vi "~sequence2.vi"(6 "i":i32, 10 "Array":T5[](array[typedef])) -> (0 "Command":string, 1 "Attenuation dB":dbl, 2 "Phase Shift deg":dbl, 3 "NewSetup":T1, 4 "Sequence is done":bool)   [LabVIEW 2017]
uses:
  Classes/Sequence/SequenceSubvis/TestStep-StepType.ctl
  Classes/Sequence/SequenceSubvis/RF Direction.ctl
  Classes/Sequence/SequenceSubvis/PolarizationSelect.ctl
  Classes/Sequence/SequenceSubvis/TestStepTypes.ctl
  Classes/Sequence/SequenceSubvis/TestStep.ctl
  Classes/Sequence/SequenceSubvis/PatchNewTestStep.ctl
panel:
  out "Test":T4
  # "This oject has members:\n- init\n- sequence\n- reset ?"
  # "NewStep\nNextPhaseShift\nNextAtten\nSequenceComplete"
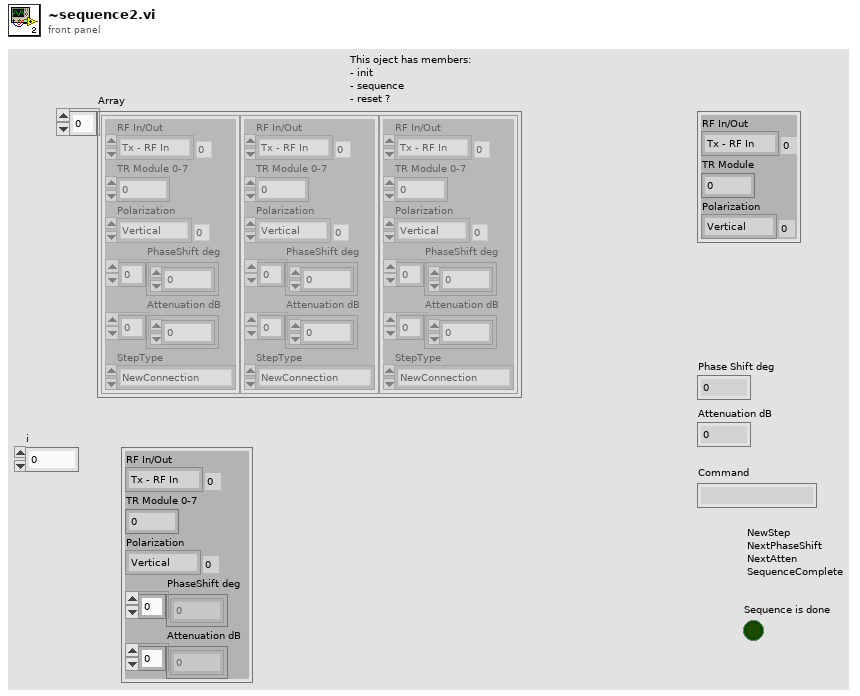
[diagram p1: front panel]
types:
  T1 = typedef "PatchNewTestStep.ctl" = cluster{"RF In/Out":T2, "TR Module":i32, "Polarization":T3}
  T2 = typedef "RF Direction.ctl" = enum16{"Tx - RF In", "Rx - RF Out"}
  T3 = typedef "PolarizationSelect.ctl" = enum16{"Vertical", "Horizontal"}
  T4 = typedef "TestStep.ctl" = cluster{"RF In/Out":T2, "TR Module 0-7":i32, "Polarization":T3, "PhaseShift deg":dbl[], "Attenuation dB":dbl[]}
  T5 = typedef "TestStep-StepType.ctl" = cluster{"RF In/Out":T2, "TR Module 0-7":i32, "Polarization":T3, "PhaseShift deg":dbl[], "Attenuation dB":dbl[], "StepType":T6}
  T6 = typedef "TestStepTypes.ctl" = enum16{"NewConnection", "SweepTest", "Motion", "Finish"}
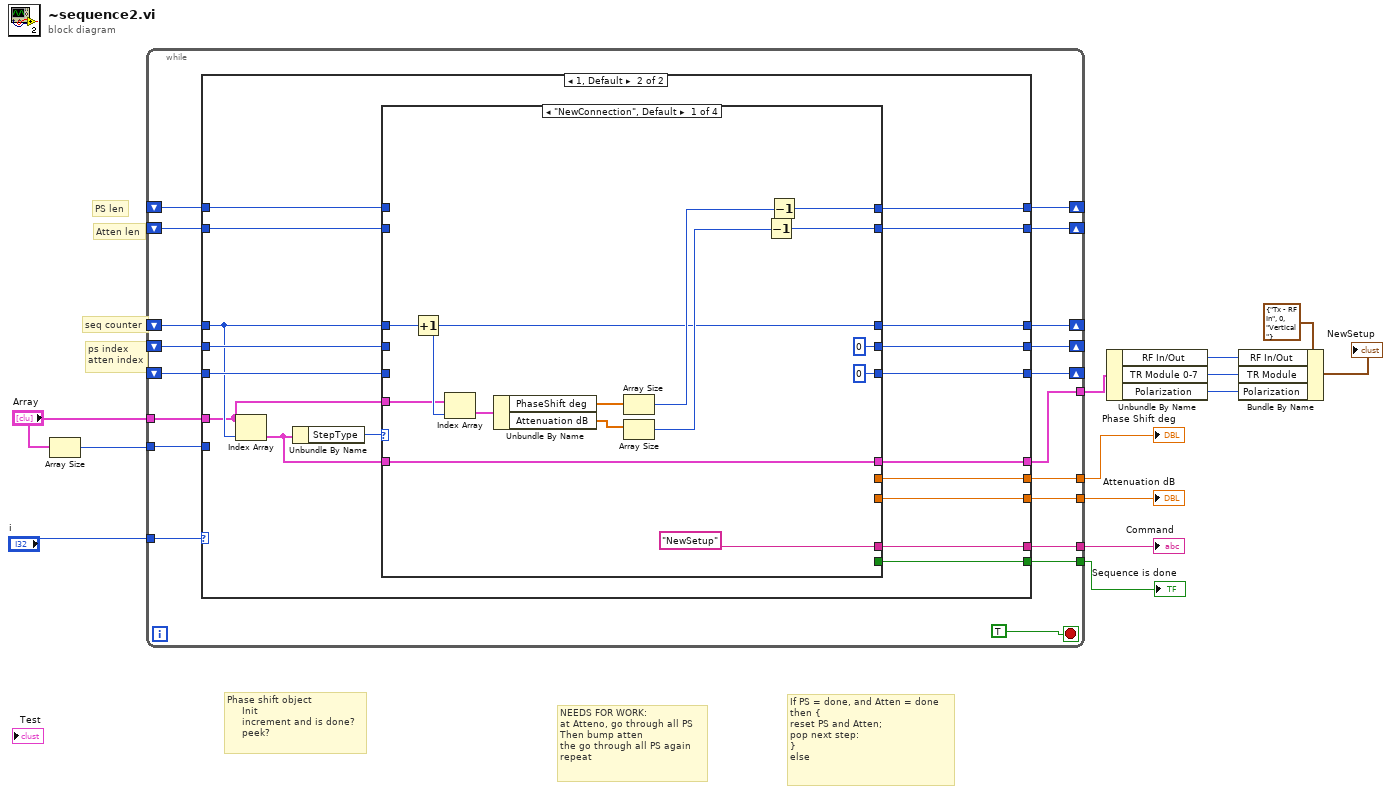
[diagram p0: block diagram]
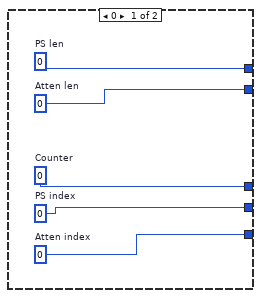
[diagram p2: hidden frame]
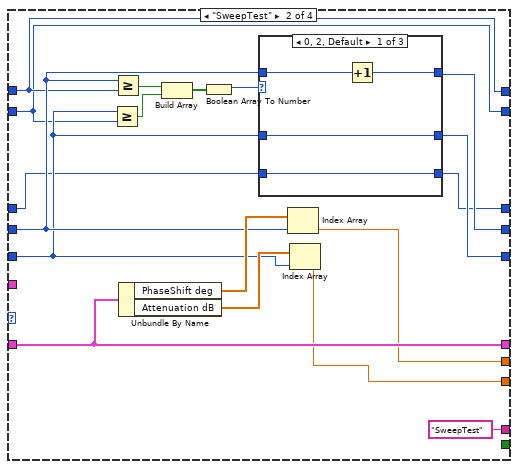
[diagram p3: hidden frame]
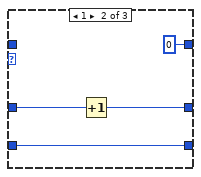
[diagram p4: hidden frame]
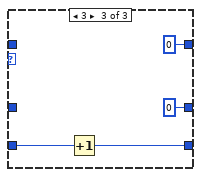
[diagram p5: hidden frame]
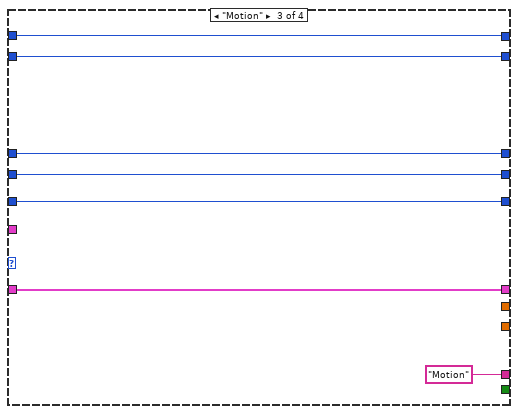
[diagram p6: hidden frame]
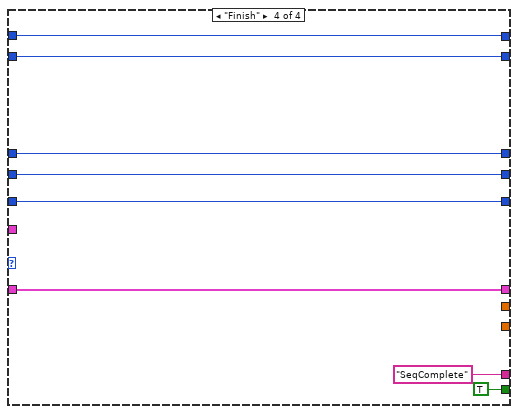
[diagram p7: hidden frame]
diagram:
  # "ps index\natten index"
  # "seq counter"
  # "Atten len"
  # "PS len"
  # "NEEDS FOR WORK:\nat Atteno, go through all PS\nThen bump atten\nthe go through all PS again\nrepeat"
  # "If PS = done, and Atten = done\nthen {\nreset PS and Atten;\npop next step:\n}\nelse"
  # "Phase shift object\n     Init\n     increment and is done?\n     peek?"
  n1 = Array Size(array="Array") -> (size(s)=w11:i32)
  n2 = while {
    shift-right: [w30] -> _
    shift-left: _ -> [w21]
    tunnel: "Array" -> [w29]
    shift-right: [w32] -> _
    shift-left: _ -> [w25]
    shift-right: [w31] -> _
    shift-left: _ -> [w24]
    shift-right: [w28] -> _
    shift-left: _ -> [w23]
    shift-right: [w27] -> _
    shift-left: _ -> [w22]
    tunnel: w11 -> [w20]
    tunnel: "i" -> [w19]
    tunnel: [w18] -> w5
    tunnel: [w17] -> w4
    tunnel: [w16] -> w3
    tunnel: [w15] -> w2
    tunnel: [w14] -> w1
    stop <- TRUE stop-if-true
    n3 = case shown="1, Default" w19 {
      tunnel: [w34 w44] -> w32
      tunnel: [w33 w45] -> w31
      tunnel: [w35 w40] -> w30
      tunnel: w29 -> [_ w38]
      tunnel: [w36 w42] -> w28
      tunnel: [w37 w43] -> w27
      tunnel: w25 -> [_ w51]
      tunnel: w24 -> [_ w50]
      tunnel: w23 -> [_ w46]
      tunnel: w22 -> [_ w47]
      tunnel: w21 -> [_ w41]
      tunnel: w20 -> [_ _]
      tunnel: [_ w53] -> w18
      tunnel: [_ w52] -> w17
      tunnel: [_ w49] -> w16
      tunnel: [_ w48] -> w15
      tunnel: [_ w39] -> w14
      frame 0 {
        w37 = 0  # PS len
        w36 = 0  # Atten len
        w33 = 0  # Atten index
        w34 = 0  # PS index
        w35 = 0  # Counter
      }
      frame 1, Default {
        n4 = Index Array(array=w38, index=w41) -> (element=w54:T5)
        n5 = Unbundle By Name(w54) -> ("StepType"=w55:T6)
        n6 = case shown="\"NewConnection\", Default" w55 {
          tunnel: w54 -> [w59 w86 w100 w108]
          tunnel: ["NewSetup" ("Command") "SweepTest" ("Command") "Motion" ("Command") "SeqComplete" ("Command")] -> w53
          tunnel: [w59 w86 w100 w108] -> w52
          tunnel: w51 -> [_ w77 w102 w110]
          tunnel: w50 -> [_ w76 w101 w109]
          tunnel: [_ w83 _ _] -> w49
          tunnel: [_ w82 _ _] -> w48
          tunnel: w47 -> [_ w73 w105 w113]
          tunnel: w46 -> [_ w72 w104 w112]
          tunnel: [0 ("Atten index") w75 w101 w109] -> w45
          tunnel: [0 w74 w102 w110] -> w44
          tunnel: [w57 w73 w105 w113] -> w43
          tunnel: [w56 w72 w104 w112] -> w42
          tunnel: w41 -> [w64 w70 w103 w111]
          tunnel: [w60 w71 w103 w111] -> w40
          tunnel: [_ _ _ TRUE] -> w39
          tunnel: w38 -> [w58 _ _ _]
          frame "NewConnection", Default {
            n7 = Increment(x=w64) -> (x+1=w60:i32)
            n8 = Index Array(array=w58, index=w60) -> (element=w61:T5)
            n9 = Unbundle By Name(w61) -> ("PhaseShift deg"=w68:dbl[], "Attenuation dB"=w67:dbl[])
            n10 = Array Size(array=w68) -> (size(s)=w66:i32)
            n11 = Array Size(array=w67) -> (size(s)=w65:i32)
            n12 = Decrement(x=w65) -> (x-1=w56:i32)
            n13 = Decrement(x=w66) -> (x-1=w57:i32)
          }
          frame "SweepTest" {
            n14 = Greater Or Equal?(x=w76, y=w72) -> (x >= y?=w80:bool)
            n15 = Greater Or Equal?(x=w77, y=w73) -> (x >= y?=w81:bool)
            n16 = Unbundle By Name(w86) -> ("PhaseShift deg"=w85:dbl[], "Attenuation dB"=w84:dbl[])
            n17 = Build Array(w81, w80) -> (w79:bool[])
            n18 = Boolean Array To Number(Boolean array=w79) -> (number=w78:u32)
            n19 = case shown="0, 2, Default" w78 {
              tunnel: [w90 0 0] -> w74
              tunnel: w77 -> [w91 _ _]
              tunnel: [w89 w93 0 ("Atten index")] -> w75
              tunnel: w76 -> [w89 w94 _]
              tunnel: w70 -> [w88 w92 w97]
              tunnel: [w88 w92 w96] -> w71
              frame 0, 2, Default {
                n20 = Increment(x=w91) -> (x+1=w90:i32)
              }
              frame 1 {
                n21 = Increment(x=w94) -> (x+1=w93:i32)
              }
              frame 3 {
                n22 = Increment(x=w97) -> (x+1=w96:i32)
              }
            }
            n23 = Index Array(array=w85, index=w77) -> (element=w82:dbl)
            n24 = Index Array(array=w84, index=w76) -> (element=w83:dbl)
          }
          frame "Motion" {
          }
          frame "Finish" {
          }
        }
      }
    }
  }
  "Command" <- w5
  "Sequence is done" <- w1
  "Phase Shift deg" <- w2
  "Attenuation dB" <- w3
  n25 = Unbundle By Name(w4) -> ("RF In/Out"=w10:T2, "TR Module 0-7"=w8:i32, "Polarization"=w7:T3)
  n26 = Bundle By Name(cluster=T1 {"RF In/Out"=enum."Tx - RF In", "TR Module"=0, "Polarization"=enum."Vertical"} ("NewSetup"), "RF In/Out"=w10, "TR Module"=w8, "Polarization"=w7) -> (→"NewSetup":T1)
